vi "Back TO.vi"(8 "error in (no error)":errorcluster, 10 "time back (ms)":u32=500, 11 "State Machine in":refnum<class "State Machine.lvclass">) -> (0 "error out":errorcluster, 3 "State Machine out":refnum<class "State Machine.lvclass">)   [LabVIEW 2018, in "State Machine.lvclass"]
uses:
  State Machine.lvclass
  State Machine.lvclass/State Machine.ctl
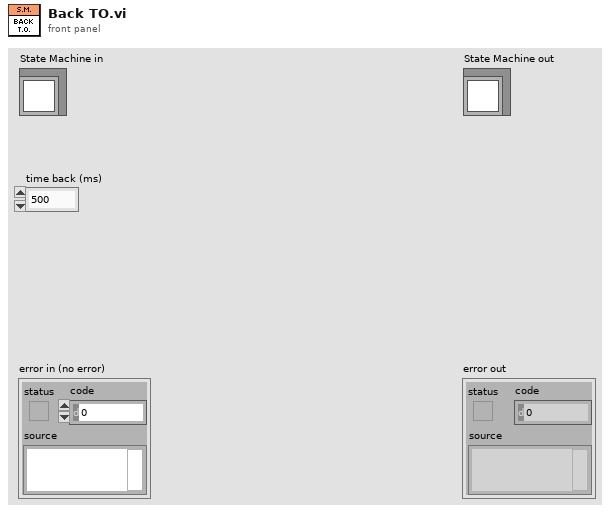
[diagram p1: front panel]
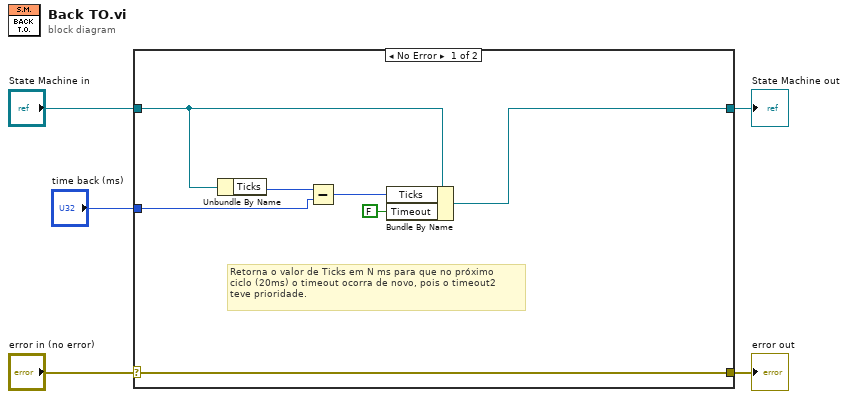
[diagram p0: block diagram]
diagram:
  n1 = case shown="No Error" "error in (no error)" {
    selector: "error in (no error)" -> [w12 w14]
    tunnel: [w12 w14] -> w4
    tunnel: [w9 w13] -> w2
    tunnel: "State Machine in" -> [w10 w13]
    tunnel: "time back (ms)" -> [w6 _]
    frame No Error {
      # "Retorna o valor de Ticks em N ms para que no próximo \nciclo (20ms) o timeout ocorra de novo, pois o timeout2 \nteve prioridade."
      n2 = Unbundle By Name(w10) -> ("Ticks"=w11:u32)
      n3 = Subtract(x=w11, y=w6) -> (x-y=w8:u32)
      n4 = Bundle By Name(cluster=w10, "Ticks"=w8, "Timeout"=FALSE) -> (w9:refnum<class "State Machine.lvclass">)
    }
    frame Error {
    }
  }
  "error out" <- w4
  "State Machine out" <- w2
